vi "Le_Finals_all.vi"() -> (0 "Data Juliana Modificada":string, 1 "Saída coord y":string, 2 "Saída coord x":string, 3 "Saída DeltaUT":string)   [LabVIEW 2018]
uses:
  Global_Telescopio.vi
panel:
  out "dia juliano":dbl format="%.6f"
  out "Coord x Rad":dbl format="%#_7f"
  out "Coord y Rad":dbl format="%#_7f"
  out "substring 3":string
  out "Coord y":dbl format="%#_7g"
  out "substring 2":string
  out "Coord x":dbl format="%#_7g"
  out "substring":string
  out "string":string
  out "Arquivo Output.txt":string
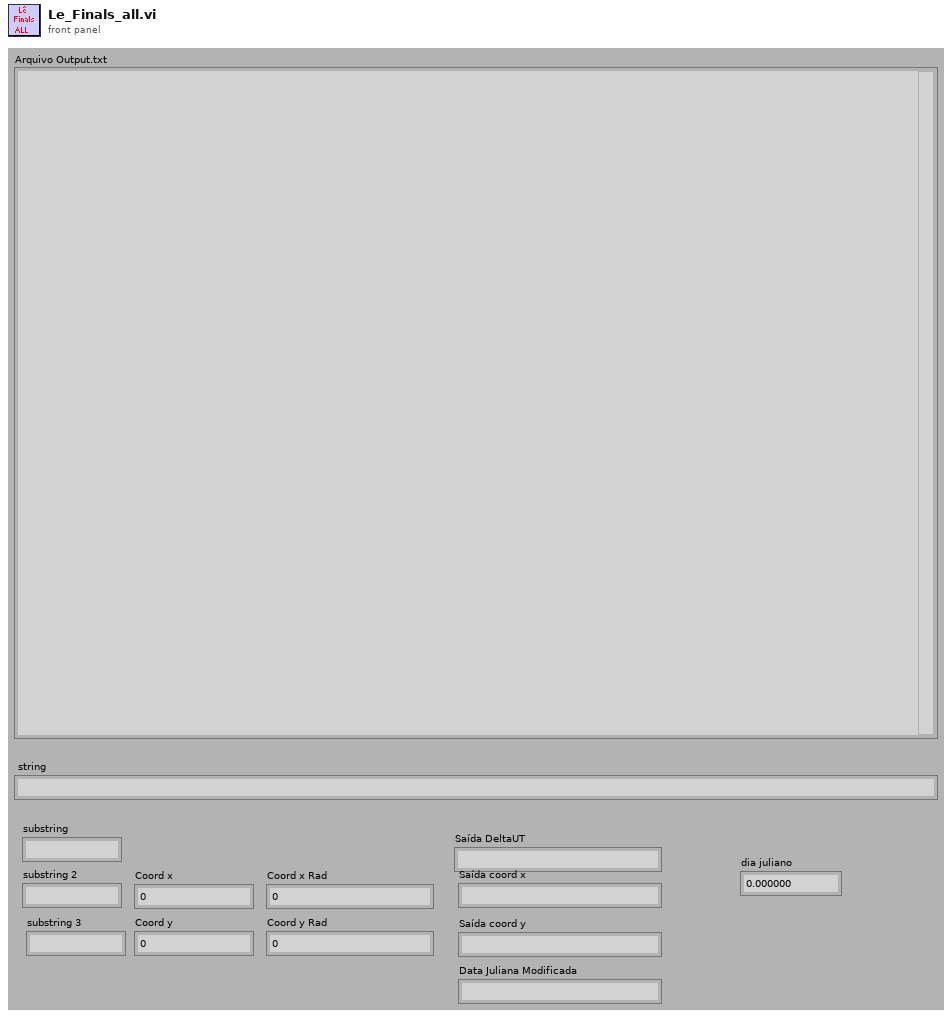
[diagram p1: front panel]
types:
  T1 = enum16{"open", "open or create", "create or replace", "create", "open (read only)"}
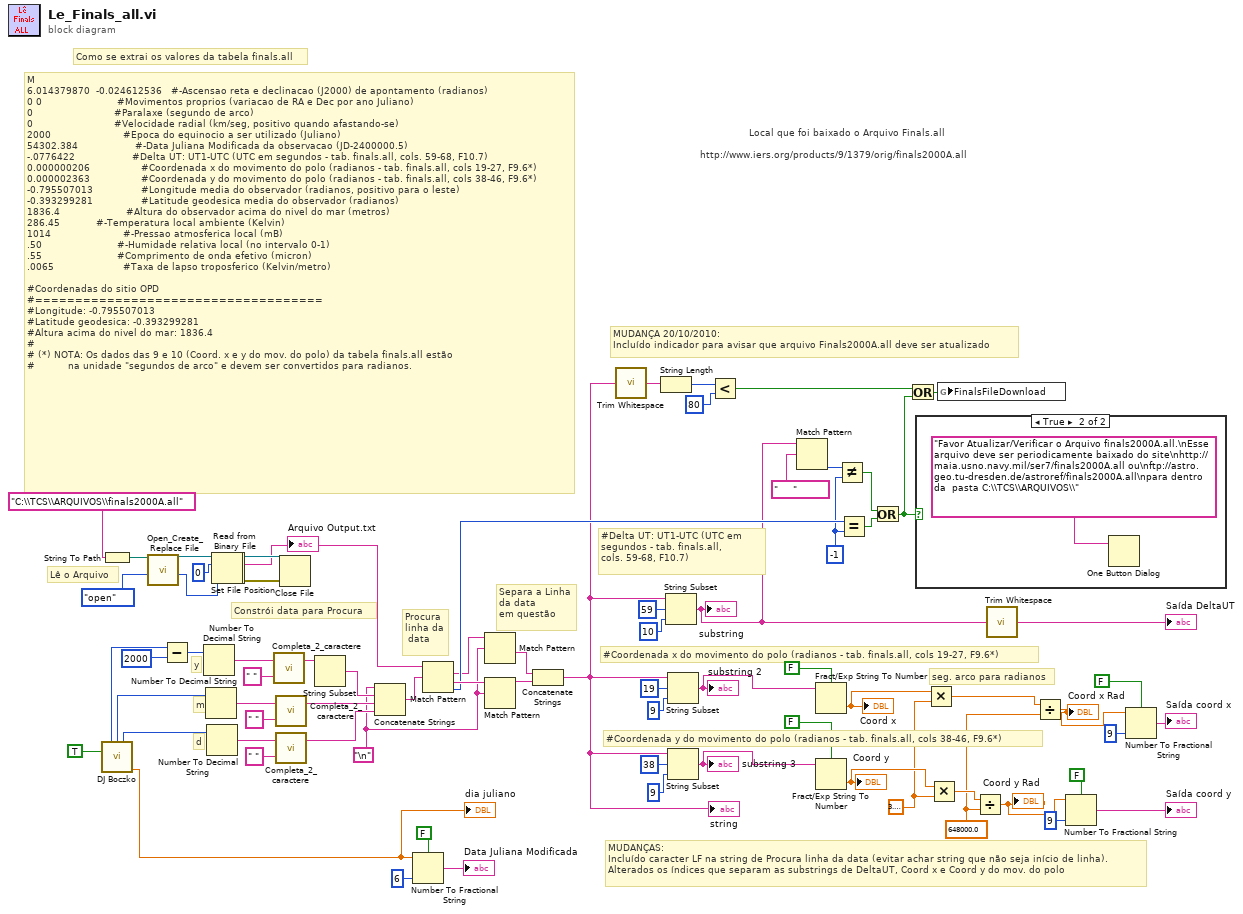
[diagram p0: block diagram]
diagram:
  w18 = "\n"
  w8 = -1 ("y")
  w12 = 648000.0 ("y")
  w13 = 3.141592653589793
  # "MUDANÇA 20/10/2010:\nIncluído indicador para avisar que arquivo Finals2000A.all deve ser atualizado"
  # "MUDANÇAS:\nIncluído caracter LF na string de Procura linha da data (evitar achar string que não seja início de linha).\nAlterados os índices que separam as substrings de DeltaUT, Coord x e Coord y do mov. do polo"
  # "Local que foi baixado o Arquivo Finals.all"
  # "http://www.iers.org/products/9/1379/orig/finals2000A.all"
  # "d"
  # "m"
  # "y"
  # "Procura\nlinha da\n data"
  # "seg. arco para radianos"
  # "#Coordenada y do movimento do polo (radianos - tab. finals.all, cols 38-46, F9.6*)"
  # "#Coordenada x do movimento do polo (radianos - tab. finals.all, cols 19-27, F9.6*)"
  # "Separa a Linha\nda data\nem questão"
  # "#Delta UT: UT1-UTC (UTC em \nsegundos - tab. finals.all, \ncols. 59-68, F10.7)"
  # "Lê o Arquivo"
  # "Constrói data para Procura"
  # "Como se extrai os valores da tabela finals.all"
  # "M\n6.014379870  -0.024612536   #-Ascensao reta e declinacao (J2000) de apontamento (radianos)\n0 0                         #Movimentos proprios (variacao de RA e Dec por ano Juliano)\n0                           #Paralaxe (segundo de arco)\n0                           #Velocidade radial (km/seg, positivo quando afastando-se)\n2000                        #Epoca do equinocio a ser utilizado (Juliano)\n54302.384                   #-Data Juliana Modificada da observacao (JD-2400000.5)\n-.0776422                   #Delta UT: UT1-UTC (UTC em segundos - tab. finals.all, cols. 59-68, F10.7)\n0.000000206                 #Coordenada x do movimento do polo (radianos - tab. finals.all, cols 19-27, F9.6*)\n0.000002363                 #Coordenada y do movimento do polo (radianos - tab. finals.all, cols 38-46, F9.6*)\n-0.795507013                #Longitude media do observador (radianos, positivo para o leste)\n-0.393299281                #Latitude geodesica media do observador (radianos)\n1836.4                      #Altura do observador acima do nivel do mar (metros)\n286.45      \t\t    #-Temperatura local ambiente (Kelvin)\n1014                        #-Pressao atmosferica local (mB)\n.50                         #-Humidade relativa local (no intervalo 0-1)\n.55                         #Comprimento de onda efetivo (micron)\n.0065                       #Taxa de lapso troposferico (Kelvin/metro)\n\n#Coordenadas do sitio OPD\n#====================================\n#Longitude: -0.795507013\n#Latitude geodesica: -0.393299281\n#Altura acima do nivel do mar: 1836.4\n#\n# (*) NOTA: Os dados das 9 e 10 (Coord. x e y do mov. do polo) da tabela finals.all estão\n#           na unidade \"segundos de arco\" e devem ser convertidos para radianos."
  n1 = String To Path(string="C:\\TCS\\ARQUIVOS\\finals2000A.all") -> (path=w11:path)
  n2 = call "DJ Boczko.vi"("TRUE = Hora Local\nFALSE = UT"=TRUE ("TRUE = Hora Local\nFALSE = UT")) -> ("ANO"=w23:i32, "MES"=w30:i32, "DIA"=w31:i32, "Dia Juliano Modificado"=w32:dbl)  [unwired: 6 in, 5 out]
  "dia juliano" <- w32
  n3 = call <vilib>:"Open_Create_Replace File.vi"("function (open:0)"=T1."open", "file path"=w11) -> ("file size (bytes)"=w72:i32, "refnum"=w73:refnum<file>)  [unwired: 6 in, 2 out]
  n4 = Subtract(x=w23, y=2000 ("length (rest)")) -> (x-y=w24:i32)
  n5 = Number To Decimal String(number=w24) -> (decimal integer string=w19:string)  [unwired: 1 in]
  n6 = Number To Decimal String(number=w30) -> (decimal integer string=w68:string)  [unwired: 1 in]
  n7 = Number To Decimal String(number=w31) -> (decimal integer string=w66:string)  [unwired: 1 in]
  n8 = Set File Position(offset (in bytes) (0)=0 ("pos offset (0)"), refnum=w73) -> (refnum out=w2:refnum<file>, error out=w1:errorcluster)  [unwired: 2 in]
  n9 = Read from Binary File(8:w1, 10:w72, 11:w2) -> (0:w75:errorcluster, 2:w62:string, 3:w76:refnum<file>)  [unwired: 3 in, 1 out]
  "Arquivo Output.txt" <- w62
  n10 = call "Completa_2_caractere.vi"("Carac para Completar"=" ", "entrada"=w19) -> ("saida"=w20:string)  [unwired: 1 in]
  n11 = call "Completa_2_caractere.vi"("Carac para Completar"=" ", "entrada"=w68) -> ("saida"=w64:string)  [unwired: 1 in]
  n12 = call "Completa_2_caractere.vi"("Carac para Completar"=" ", "entrada"=w66) -> ("saida"=w63:string)  [unwired: 1 in]
  n13 = Close File(refnum=w76, error in=w75) -> ()  [unwired: 2 out]
  n14 = String Subset(string=w20) -> (substring=w65:string)  [unwired: 2 in]
  n15 = Concatenate Strings(w18, w65, w64, w63) -> (w60:string)
  n16 = Number To Fractional String(use system decimal point (T)=FALSE, number=w32, precision (6)=i16 6) -> (F-format string=→"Data Juliana Modificada":string)  [unwired: 1 in]
  n17 = Match Pattern(string=w62, regular expression=w60) -> (match substring=w17:string, after substring=w61:string, offset past match=w25:i32)  [unwired: 1 in, 1 out]
  n18 = Match Pattern(string=w17, regular expression=w18) -> (after substring=w16:string)  [unwired: 1 in, 3 out]
  n19 = Match Pattern(string=w61, regular expression=w18) -> (before substring=w59:string)  [unwired: 1 in, 3 out]
  n20 = Concatenate Strings(w16, w59) -> (w9:string)
  "string" <- w9
  n21 = call <vilib>:"Trim Whitespace.vi"("string"=w9) -> ("trimmed string"=w10:string)  [unwired: 1 in]
  n22 = String Length(string=w10) -> (length=w6:i32)
  n23 = String Subset(string=w9, offset (0)=59, length (rest)=10 ("length (rest)")) -> (substring=w15:string)
  "substring" <- w15
  n24 = String Subset(string=w9, offset (0)=19, length (rest)=9 ("length (rest)")) -> (substring=w44:string)
  "substring 2" <- w44
  n25 = String Subset(string=w9, offset (0)=38, length (rest)=9 ("length (rest)")) -> (substring=w43:string)
  "substring 3" <- w43
  n26 = Less?(x=w6, y=80 ("offset (0)")) -> (x < y?=w3:bool)
  n27 = Match Pattern(string=w15, regular expression="     " ("y")) -> (offset past match=w28:i32)  [unwired: 1 in, 3 out]
  n28 = Fract/Exp String To Number(use system decimal point (T)=FALSE, string=w44) -> (number=w52:dbl)  [unwired: 2 in, 1 out]
  "Coord x" <- w52
  n29 = Fract/Exp String To Number(use system decimal point (T)=FALSE, string=w43) -> (number=w49:dbl)  [unwired: 2 in, 1 out]
  "Coord y" <- w49
  n30 = Not Equal?(x=w28, y=w8) -> (x != y?=w27:bool)
  n31 = Equal?(x=w25, y=w8) -> (x = y?=w26:bool)
  n32 = Or(x=w27, y=w26) -> (x .or. y?=w4:bool)
  n33 = Or(x=w3, y=w4) -> (x .or. y?=w5:bool)
  n34 = case shown="True" w4 {
    frame False {
    }
    frame True {
      n35 = One Button Dialog(message="Favor Atualizar/Verificar o Arquivo finals2000A.all.\nEsse arquivo deve ser periodicamente baixado do site\nhttp://maia.usno.navy.mil/ser7/finals2000A.all ou\nftp://astro.geo.tu-dresden.de/astroref/finals2000A.all\npara dentro da  pasta C:\\TCS\\ARQUIVOS\\") -> ()  [unwired: 1 in, 1 out]
    }
  }
  n36 = Multiply(x=w52, y=w13) -> (x*y=w51:dbl)
  n37 = Multiply(x=w49, y=w13) -> (x*y=w50:dbl)
  n38 = global write "Global_Telescopio.vi" "FinalsFileDownload"(w5) -> ()
  n39 = Divide(x=w50, y=w12) -> (x/y=w47:dbl)
  "Coord y Rad" <- w47
  n40 = call <vilib>:"Trim Whitespace.vi"("string"=w15) -> ("trimmed string"=→"Saída DeltaUT":string)  [unwired: 1 in]
  n41 = Divide(x=w51, y=w12) -> (x/y=w48:dbl)
  "Coord x Rad" <- w48
  n42 = Number To Fractional String(use system decimal point (T)=FALSE, number=w47, precision (6)=i16 9) -> (F-format string=→"Saída coord y":string)  [unwired: 1 in]
  n43 = Number To Fractional String(use system decimal point (T)=FALSE, number=w48, precision (6)=i16 9) -> (F-format string=→"Saída coord x":string)  [unwired: 1 in]
